vi "test FFT.vi"() -> ()   [LabVIEW 2013]
uses:
  <vilib>/measure/maspectr.llb/Power Spectrum and PSD Export Mode.ctl
  <vilib>/DAQmx/read.llb/DAQmx Read (Analog Wfm 1Chan NSamp).vi
  <vilib>/Analysis/2dsp.llb/Real FFT.vi
  <vilib>/Analysis/2dsp.llb/Power Spectrum (DBL).vi
  <vilib>/DAQmx/create/channels.llb/DAQmx Create Channel (AI-Voltage-Basic).vi
  <vilib>/DAQmx/configure/timing.llb/DAQmx Timing (Sample Clock).vi
  <vilib>/DAQmx/miscellaneous.llb/DAQmx Fill In Error Info.vi
  <vilib>/express/express analysis/Spectral/Block/exnSpectralBlock spectral measurements power poly.vi
  <vilib>/express/express analysis/Spectral/Block/exnSpectralBlock spectral measurements power WFM.vi
  <vilib>/measure/maspectr.llb/FFT Power Spectrum and PSD for 1 Chan.vi
  <vilib>/measure/maspectr.llb/FFT Spectrum (Mag-Phase) for 1 Chan.vi
  <vilib>/measure/maspectr.llb/FFT Spectrum (Real-Im) for 1 Chan.vi
  <vilib>/express/express analysis/Spectral/XNode/ExpressSpectralMeasurementsBlockNode.xnode
  <vilib>/Analysis/NI_AALPro.lvlib
  <vilib>/measure/NI_MAPro.lvlib
panel:
  out "Mean (DC)":dbl
  out "Waveform Graph":cluster{"f0":dbl, "df":dbl, "magnitude":dbl[]}(graph)
  out "element":string
  in  "index (row)":i32
  in  "spectrum units table":string[][](table)=[["FFT", "N * V", "N/2 * Vpk"], ["Power Spectrum", "V^2", "1/2 * Vrms^2"], ["Auto Power Spectrum", "V^2", "Vrms^2"], ["Amplitude and Phase Spectrum", "V", "Vrms"], ["FFT Power Spectrum", "V^2", "Vrms^2"], ["FFT Power Spectral Density", "V^2/Hz", "Vrms^2/Hz"], ["FFT Spectrum (Mag-Phase)", "V", "Vrms"], ["FFT Spectrum (Real-Imag)", "V", "Vrms"]]
  in  "stop":bool
  out "phase spectrum":dbl[](array[numeric])
  out "spectral plot":cluster{"t":dbl, "t":dbl, "magnitude":dbl[]}(graph)={"t"=0.0, "t"=1.0, "magnitude"=[]}
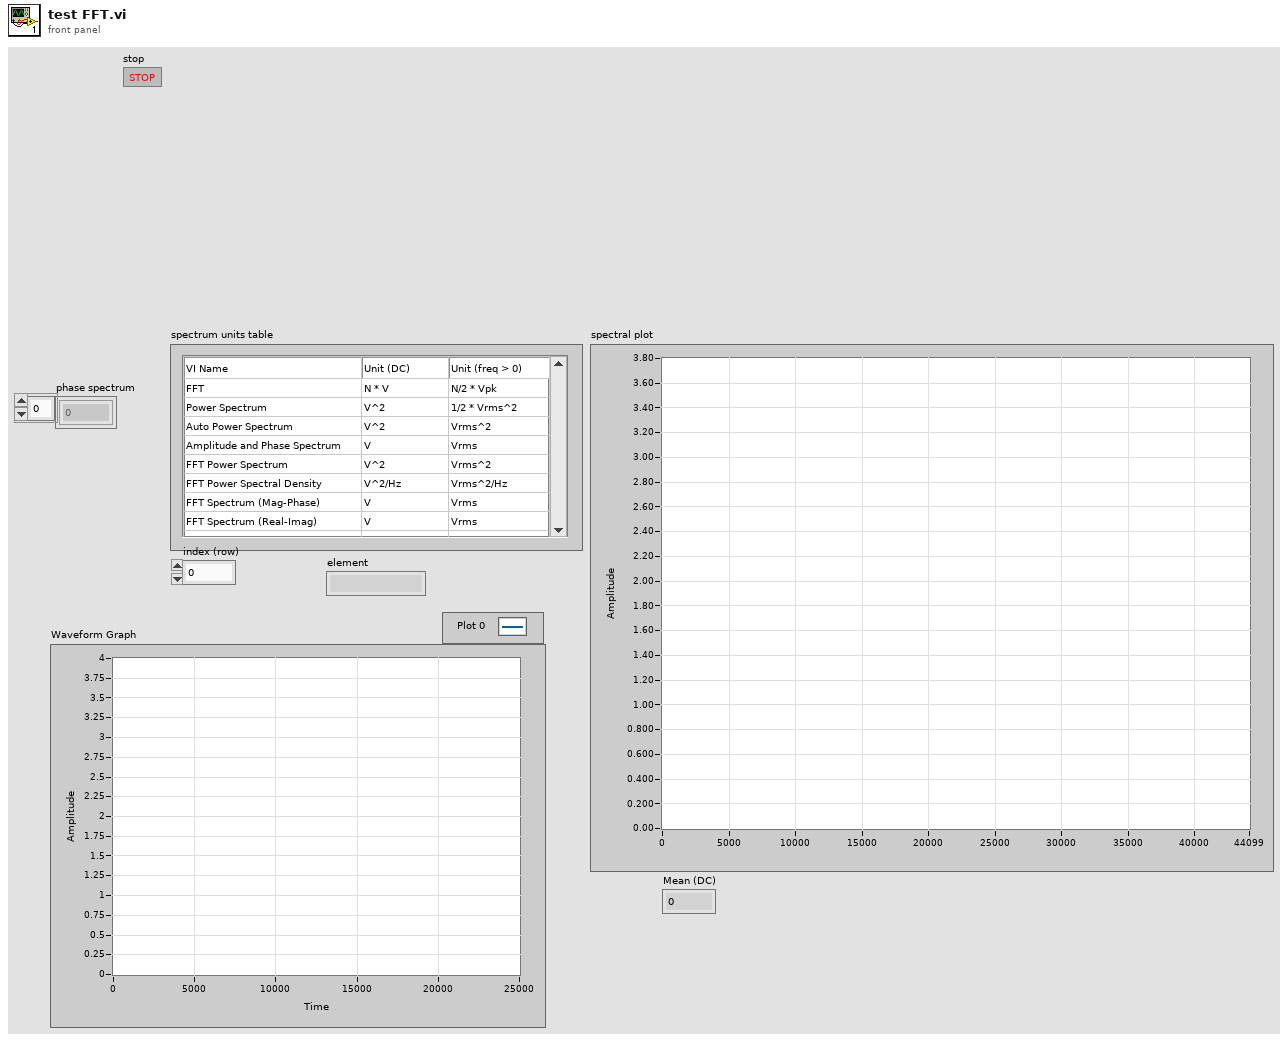
[diagram p1: front panel]
types:
  T1 = cluster{"averaging mode":u16, "weighting mode":u16, "number of averages":u32}
  T2 = cluster{"dB On (F)":bool, "unwrap phase (F)":bool, "convert to degree (F)":bool}
  T3 = enum16{"None ", "Hanning", "Hamming", "Blackman-Harris", "Exact Blackman", "Blackman", "Flat Top", "4 Term B-Harris ", "7 Term B-Harris", "Low Sidelobe"}
  T4 = typedef "NI_MAPro.lvlib/Power Spectrum and PSD Export Mode.ctl" = u16
  T5 = cluster{"f0":dbl, "df":dbl, "imaginary part":dbl[]}
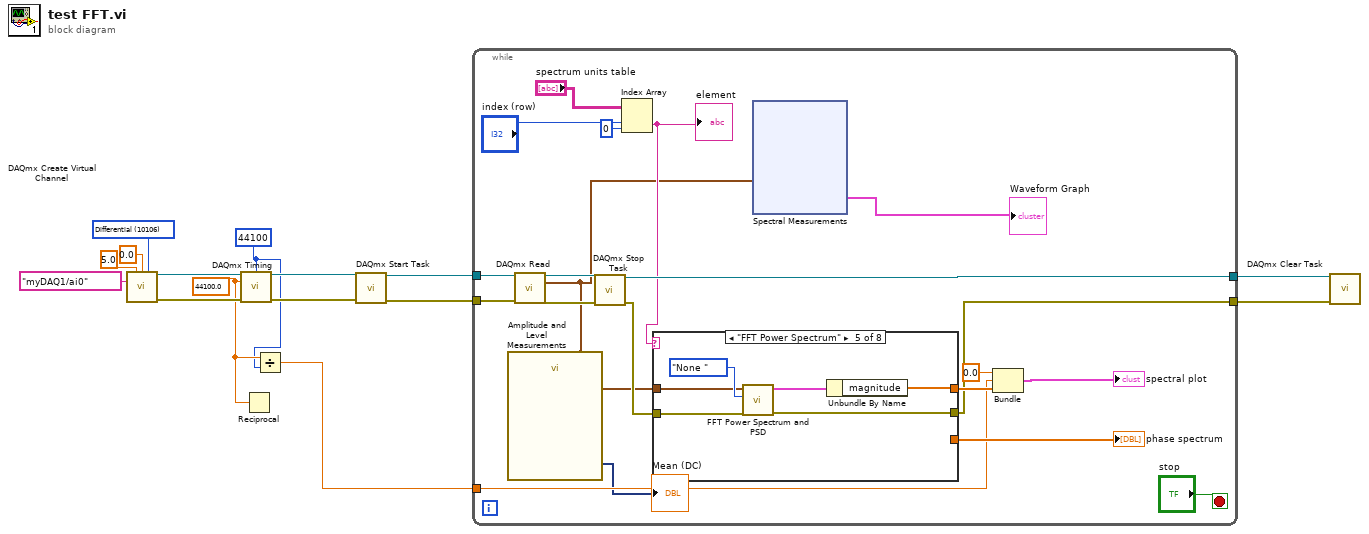
[diagram p0: block diagram]
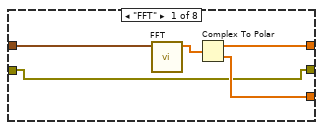
[diagram p2: hidden frame]
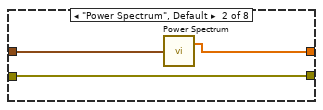
[diagram p3: hidden frame]
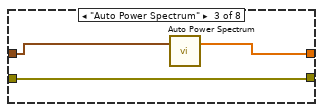
[diagram p4: hidden frame]
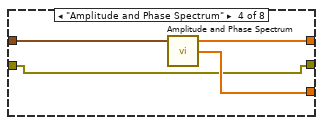
[diagram p5: hidden frame]
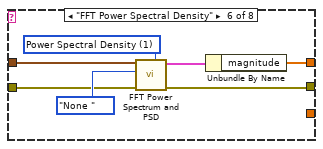
[diagram p6: hidden frame]
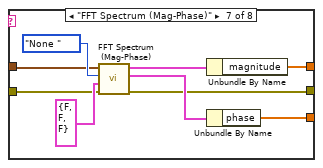
[diagram p7: hidden frame]
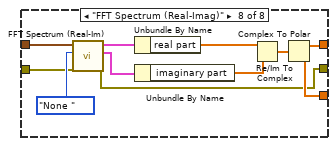
[diagram p8: hidden frame]
diagram:
  w3 = 44100.0 ("rate")
  w2 = 44100 ("samples per channel")
  w12 = 10106 items=["default"=-1, "RSE"=10083, "NRSE"=10078, "Differential"=10106, "Pseudodifferential"=12529] ("input terminal configuration")
  n1 = call-poly <vilib>:"DAQmx Create Virtual Channel.vi"("maximum value"=5.0, "minimum value"=0.0, "input terminal configuration"=w12, "physical channels"=tag "myDAQ1/ai0") -> ("task out"=w11:refnum<k21>, "error out"=w10:errorcluster)  [unwired: 5 in, 5 out]
  n2 = call-poly <vilib>:"DAQmx Timing.vi"("task/channels in"=w11, "samples per channel"=w2, "rate"=w3, "error in"=w10) -> ("task out"=w9:refnum<k21>, "error out"=w8:errorcluster)  [unwired: 3 in, 7 out]
  n3 = Reciprocal(x=w3) -> ()  [unwired: 1 out]
  n4 = Divide(x=w3, y=w2) -> (x/y=w1:dbl)
  n5 = call <vilib>:"DAQmx Start Task.vi"("task/channels in"=w9, "error in"=w8) -> ("task out"=w6:refnum<k21>, "error out"=w7:errorcluster)  [unwired: 12 out]
  n6 = while {
    tunnel: w7 -> [w33]
    tunnel: w6 -> [w32]
    tunnel: [w31] -> w4
    tunnel: [w24] -> w5
    tunnel: w1 -> [w26]
    stop <- "stop" stop-if-true
    n7 = call-poly <vilib>:"DAQmx Read.vi"("task/channels in"=w32, "error in"=w33) -> ("task out"=w35:refnum<k21>, "data"=w17:waveform(dbl), "error out"=w34:errorcluster)  [unwired: 1 in, 10 out]
    n8 = call "Amplitude and Level Measurements"("Signals"=w17) -> ("Mean (DC)"=→"Mean (DC)":dynamicdata)  [unwired: 13 in, 1 out]
    n9 = call <vilib>:"DAQmx Stop Task.vi"("task/channels in"=w35, "error in"=w34) -> ("task out"=w31:refnum<k21>, "error out"=w25:errorcluster)  [unwired: 12 out]
    n10 = Index Array(array="spectrum units table", index (row)="index (row)", index (col)=0 ("disabled index (col)")) -> (element=w19:string)
    "element" <- w19
    n11 = case shown="\"FFT Power Spectrum\"" w19 {
      tunnel: [w48 w52 w55 w59 w64 w71 w80 w86] -> w29
      tunnel: [w47 _ _ w58 _ _ w77 w85] -> w27
      tunnel: [w45 w50 w53 w56 w62 w68 w75 w84] -> w24
      tunnel: w17 -> [w46 w51 w54 w57 w61 w67 w73 w83]
      tunnel: w25 -> [w45 w50 w53 w56 w60 w66 w74 w82]
      frame "FFT" {
        n12 = call-poly <vilib>:"FFT.vi"("X"=w46) -> ("FFT {X}"=w49:cdb[])  [unwired: 9 in, 1 out]
        n13 = Complex To Polar(r * e^(i*theta)=w49) -> (r=w48:dbl[], theta=w47:dbl[])
      }
      frame "Power Spectrum", Default {
        n14 = call-poly <vilib>:"Power Spectrum.vi"("X"=w51) -> ("Power Spectrum"=w52:dbl[])  [unwired: 1 out]
      }
      frame "Auto Power Spectrum" {
        n15 = call <vilib>:"Auto Power Spectrum.vi"("Signal (V)"=w54) -> ("Power Spectrum (V^2 rms)"=w55:dbl[])  [unwired: 1 in, 1 out]
      }
      frame "Amplitude and Phase Spectrum" {
        n16 = call <vilib>:"Amplitude and Phase Spectrum.vi"("Signal (V)"=w57) -> ("Amp Spectrum Phase (radians)"=w58:dbl[], "Amp Spectrum Mag (Vrms)"=w59:dbl[])  [unwired: 2 in, 1 out]
      }
      frame "FFT Power Spectrum" {
        n17 = call-poly <vilib>:"FFT Power Spectrum and PSD.vi"("error in (no error)"=w60, "window"=T3."None ", "time signal"=w61) -> ("error out"=w62:errorcluster, "Power Spectrum / PSD"=w65:cluster{"f0":dbl, "df":dbl, "magnitude":dbl[]})  [unwired: 5 in, 2 out]
        n18 = Unbundle By Name(w65) -> ("magnitude"=w64:dbl[])
      }
      frame "FFT Power Spectral Density" {
        w69 = T4 1 items=["Power Spectrum", "Power Spectral Density"] ("export mode")
        n19 = call-poly <vilib>:"FFT Power Spectrum and PSD.vi"("export mode"=w69, "error in (no error)"=w66, "window"=T3."None ", "time signal"=w67) -> ("error out"=w68:errorcluster, "Power Spectrum / PSD"=w72:cluster{"f0":dbl, "df":dbl, "magnitude":dbl[]})  [unwired: 4 in, 2 out]
        n20 = Unbundle By Name(w72) -> ("magnitude"=w71:dbl[])
      }
      frame "FFT Spectrum (Mag-Phase)" {
        n21 = call-poly <vilib>:"FFT Spectrum (Mag-Phase).vi"("error in (no error)"=w74, "view"=T2 {"dB On (F)"=FALSE, "unwrap phase (F)"=FALSE, "convert to degree (F)"=FALSE}, "window"=T3."None ", "time signal"=w73) -> ("error out"=w75:errorcluster, "phase"=w78:cluster{"f0":dbl, "df":dbl, "phase":dbl[]}, "magnitude"=w81:cluster{"f0":dbl, "df":dbl, "magnitude":dbl[]})  [unwired: 3 in, 2 out]
        n22 = Unbundle By Name(w81) -> ("magnitude"=w80:dbl[])
        n23 = Unbundle By Name(w78) -> ("phase"=w77:dbl[])
      }
      frame "FFT Spectrum (Real-Imag)" {
        n24 = call-poly <vilib>:"FFT Spectrum (Real-Im).vi"("error in (no error)"=w82, "window"=T3."None ", "time signal"=w83) -> ("error out"=w84:errorcluster, "imaginary part"=w90:T5, "real part"=w92:cluster{"f0":dbl, "df":dbl, "real part":dbl[]})  [unwired: 4 in, 2 out]
        n25 = Unbundle By Name(w92) -> ("real part"=w89:dbl[])
        n26 = Unbundle By Name(w90) -> ("imaginary part"=w88:dbl[])
        n27 = Re/Im To Complex(1:w88, 2:w89) -> (0:w87:cdb[])
        n28 = Complex To Polar(r * e^(i*theta)=w87) -> (r=w86:dbl[], theta=w85:dbl[])
      }
    }
    "phase spectrum" <- w27
    n29 = xnode "Spectral Measurements"("Signals"=w17) -> ("Power Spectrum"=→"Waveform Graph":cluster{"f0":dbl, "df":dbl, "magnitude":dbl[]})  [unwired: 1 in, 1 out]
    n30 = Bundle("t"=0.0, w26, "magnitude"=w29) -> (→"spectral plot":cluster{"t":dbl, dbl, "magnitude":dbl[]})  [unwired: 1 in]
  }
  n31 = call <vilib>:"DAQmx Clear Task.vi"("task in"=w4, "error in"=w5) -> ()  [unwired: 13 in, 1 out]
